vi "HandsOnCfgUI.vi"() -> ()   [LabVIEW 2013]
uses:
  <vilib>/NI/Tag Bus Data Framework/Configuration Editor/Classes/Engine Parent/Engine Parent Editor Node.lvclass
  <vilib>/NI/Tag Bus Data Framework/Configuration Editor/Classes/Module editor node/module editor node.lvclass
  <vilib>/NI/Tag Bus Data Framework/control module/editor node/control module editor.lvclass
  <vilib>/NI/Tools/Keyed Array/KeyedArray.ctl
  <vilib>/NI/Tools/Keyed Array/Tools_KeyedArray.lvlib
  <vilib>/NI/AMC/Message.ctl
  <vilib>/NI/AMC/AMC.lvlib
  <vilib>/NI/AMC/Message Queue.ctl
  <vilib>/NI/Configuration Framework/Node/NISE_CEF_Node.lvclass
  <vilib>/NI/Configuration Framework/Node/NodeRef.ctl
  <vilib>/NI/Configuration Framework/Controls/EventCluster.ctl
  <vilib>/NI/Configuration Framework/NISE_CEF_TreeControl.lvlib
  <vilib>/NI/Configuration Framework/Node/UserEventRef.ctl
  <vilib>/NI/Configuration Framework/Node/RefreshUIEvent.ctl
  <vilib>/NI/Configuration Framework/Node/CacheState.ctl
  <vilib>/NI/Configuration Framework/Node/StopEvent.ctl
  <vilib>/NI/Configuration Framework/Node/NodeChangeEvent.ctl
panel:
  in  "output range low":dbl
  in  "output range high":dbl
  in  "Output mappings":cluster{"fan":string, "lamp":string}
  in  "Input mappings":T1
  in  "node change":T2
  in  "stop event":T3
  in  "cache state":T4
  in  "refresh UI":T5
  in  "user event":T6
  in  "main queue":T7
  in  "node ref":T8
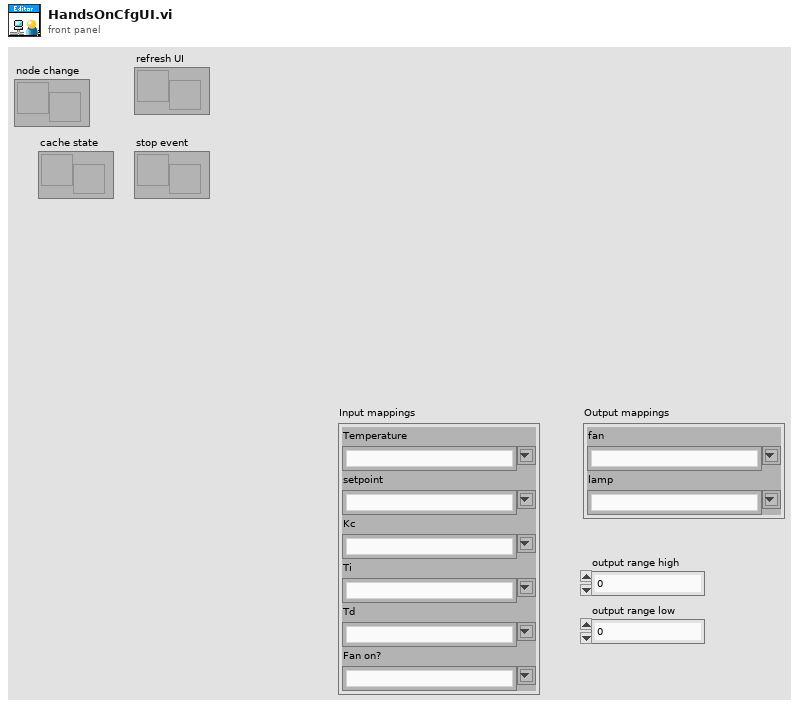
[diagram p1: front panel]
types:
  T1 = cluster{"Temperature":string, "setpoint":string, "Kc":string, "Ti":string, "Td":string, "Fan on?":string}
  T2 = typedef "NISE_CEF_Node.lvclass/NodeChangeEvent.ctl" = refnum<user-event>
  T3 = typedef "NISE_CEF_Node.lvclass/StopEvent.ctl" = refnum<user-event>
  T4 = typedef "NISE_CEF_Node.lvclass/CacheState.ctl" = refnum<user-event>
  T5 = typedef "NISE_CEF_Node.lvclass/RefreshUIEvent.ctl" = refnum<user-event>
  T6 = typedef "NISE_CEF_Node.lvclass/UserEventRef.ctl" = refnum<user-event>
  T7 = typedef "AMC.lvlib/Message Queue.ctl" = refnum<queue>
  T8 = typedef "NISE_CEF_Node.lvclass/NodeRef.ctl" = refnum<data-value>
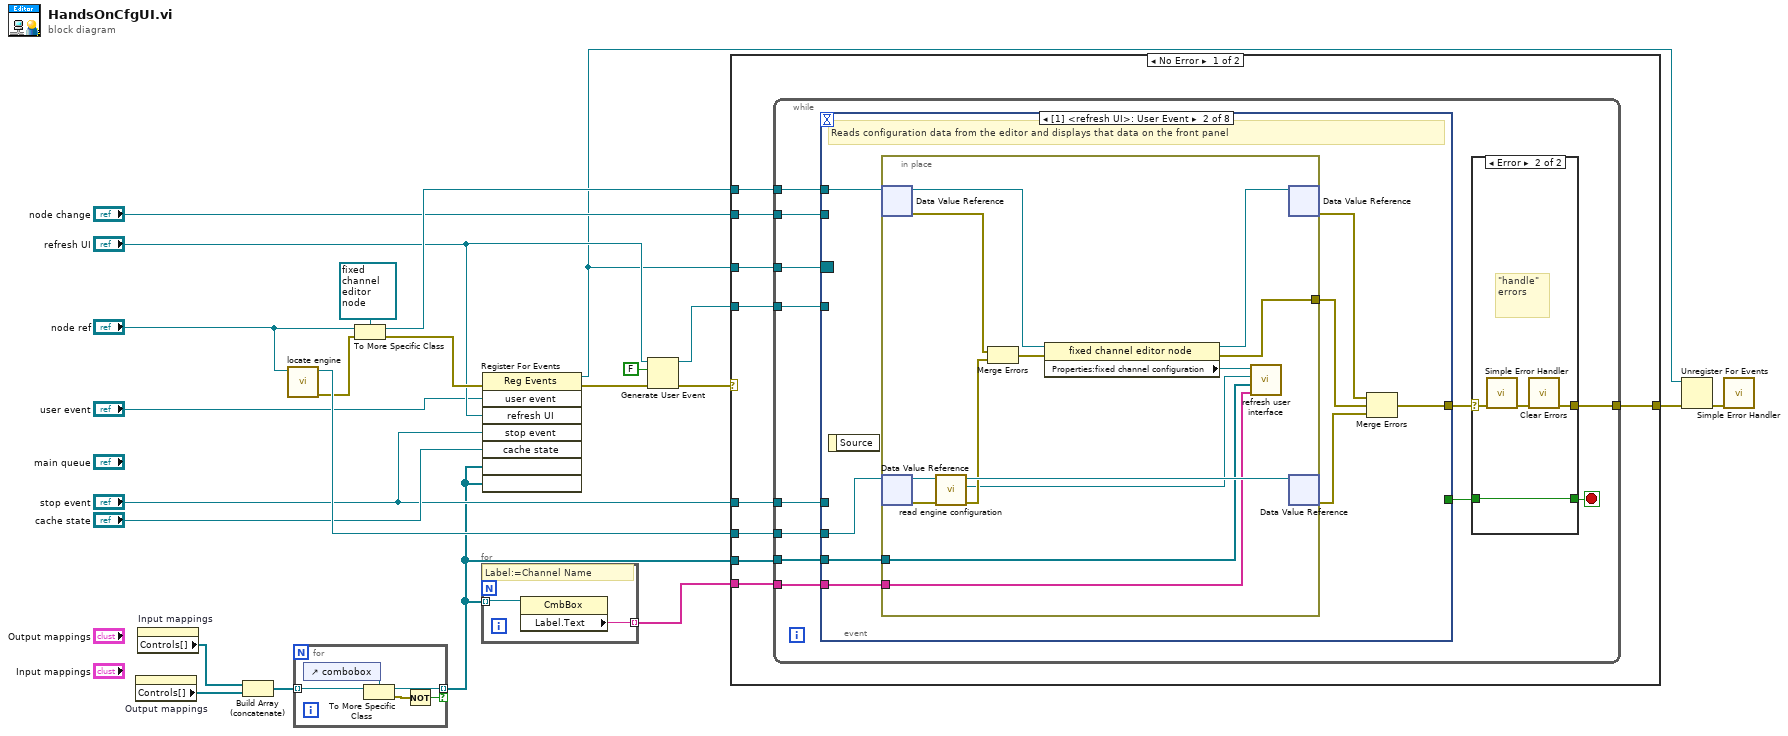
[diagram p0: block diagram]
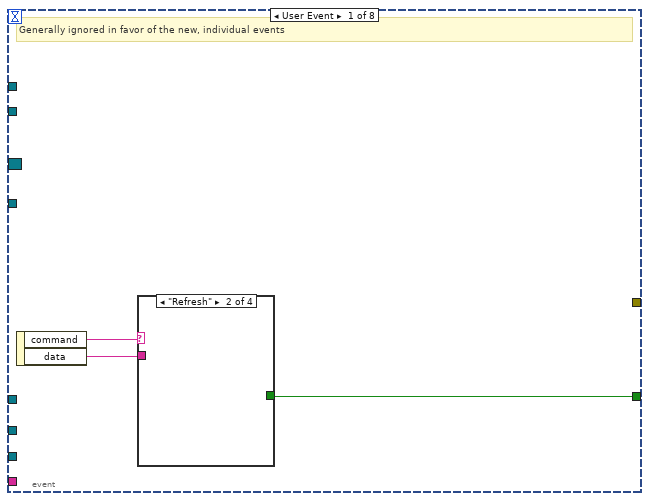
[diagram p3: hidden frame]
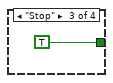
[diagram p5: hidden frame]
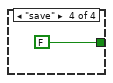
[diagram p6: hidden frame]
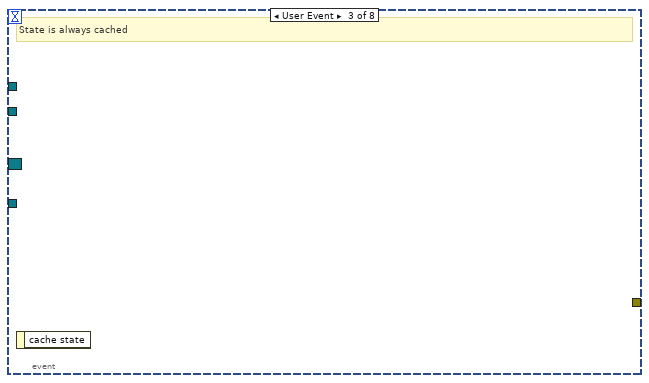
[diagram p7: hidden frame]
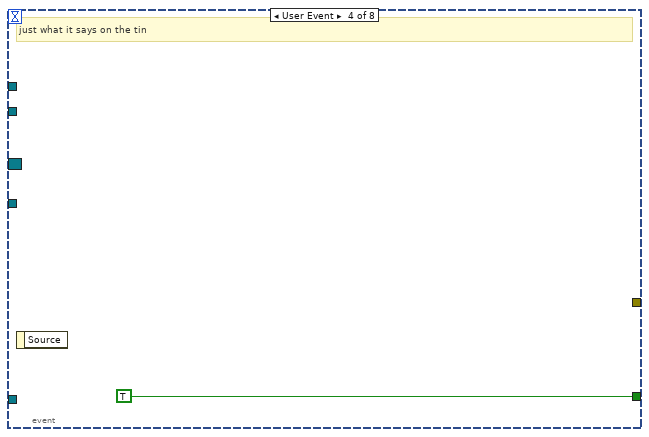
[diagram p8: hidden frame]
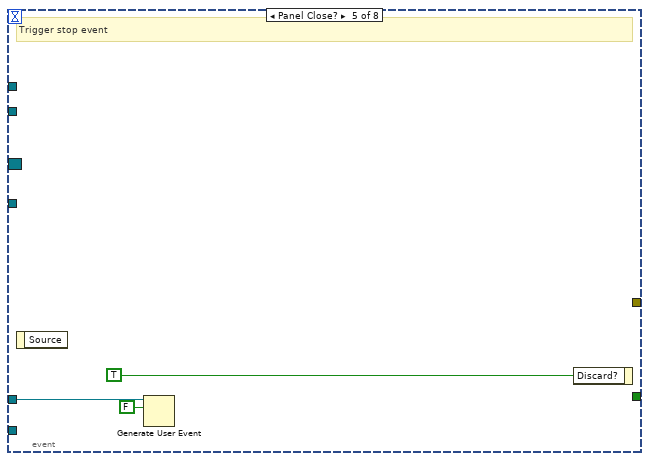
[diagram p9: hidden frame]
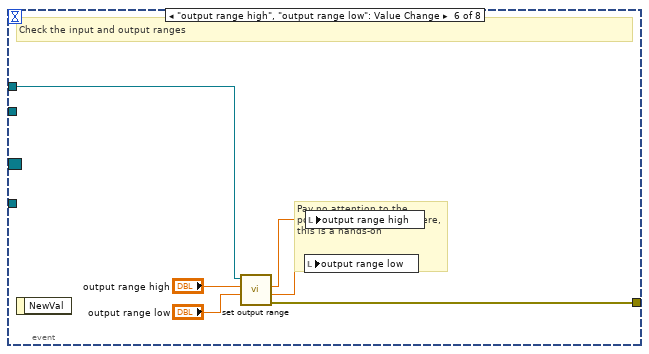
[diagram p10: hidden frame]
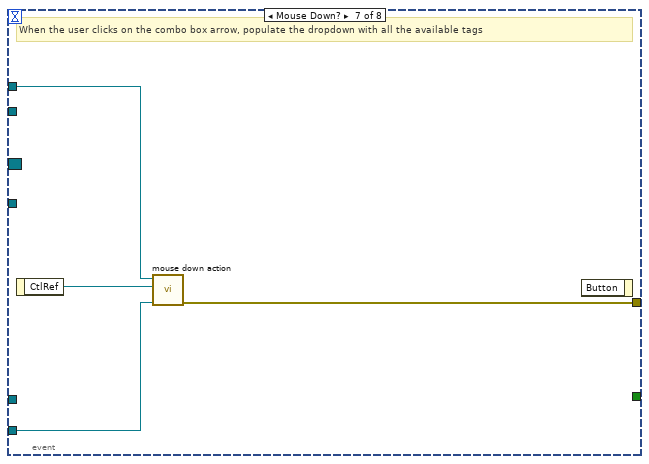
[diagram p11: hidden frame]
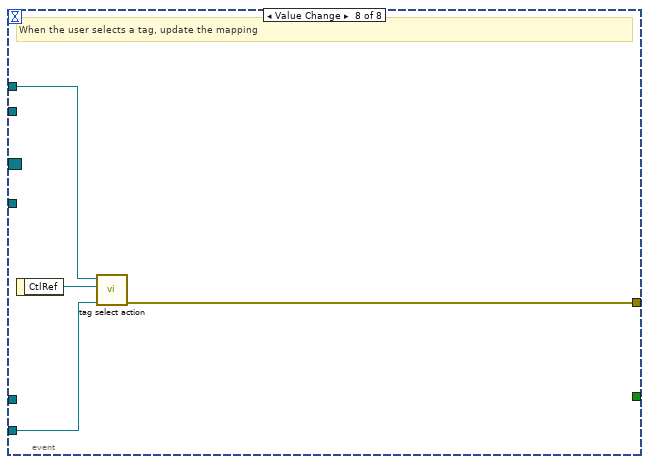
[diagram p12: hidden frame]
diagram:
  n1 = property on="Output mappings" class="Clust (strict)"() -> ("Controls[]"=w5:refnum<vi>[])  [unwired: 2 in, 2 out]
  n2 = property on="Input mappings" class="Clust (strict)"() -> ("Controls[]"=w6:refnum<vi>[])  [unwired: 2 in, 2 out]
  n3 = Build Array (concatenate)(w6, w5) -> (w3:refnum<vi>[])
  n4 = call <vilib>:"locate engine.vi"("component"="node ref") -> ("error out"=w15:errorcluster, "engine"=w17:refnum<data-value>)  [unwired: 9 in]
  n5 = for {
    tunnel: [w27] -> w1 mode=indexing if=w25
    tunnel: w3 -> [w28] mode=indexing
    n6 = control-ref of="combobox"() -> (w24:refnum<vi>)
    n7 = To More Specific Class(target class=w24, reference=w28) -> (specific class reference=w27:refnum<vi>, error out=w26:errorcluster)  [unwired: 1 in]
    n8 = Not(x=w26) -> (.not. x?=w25:bool)
  }
  n9 = To More Specific Class(target class=refnum<data-value> refnum ("data value reference"), reference="node ref", error in=w15) -> (specific class reference=w19:refnum<data-value>, error out=w18:errorcluster)
  n10 = for {
    tunnel: [w30] -> w4 mode=indexing
    tunnel: w1 -> [w29] mode=indexing
    # "Label:=Channel Name"
    n11 = property class="CmbBox"(reference=w29) -> ("Label.Text"=w30:string)  [unwired: 1 in, 2 out]
  }
  n12 = register-events(error in=w18, "user event", "refresh UI", "stop event", "cache state", w1, w1) -> (reference out=w2:refnum<event-registration>, error out=w21:errorcluster)  [unwired: 1 in]
  n13 = Generate User Event(user event="refresh UI", event data cluster=FALSE ("event data"), error in=w21) -> (user event out=w10:T5, error out=w14:errorcluster)  [unwired: 1 in]
  n14 = case shown="No Error" w14 {
    selector: w14 -> [_ w102]
    tunnel: w2 -> [w39 _]
    tunnel: [w36 w102] -> w23
    tunnel: w17 -> [w38 _]
    tunnel: w19 -> [w37 _]
    tunnel: "node change" -> [w35 _]
    tunnel: w10 -> [w34 _]
    tunnel: "stop event" -> [w33 _]
    tunnel: w1 -> [w32 _]
    tunnel: w4 -> [w31 _]
    frame No Error {
      n15 = while {
        tunnel: w39 -> [w51]
        tunnel: w37 -> [w48]
        tunnel: w38 -> [w47]
        tunnel: [w45] -> w36
        tunnel: w35 -> [w44]
        tunnel: w34 -> [w43]
        tunnel: w33 -> [w42]
        tunnel: w32 -> [w41]
        tunnel: w31 -> [w40]
        stop <- w49 stop-if-true
        n16 = event shown="[1] <refresh UI>: User Event" {
          selector: w51 -> [_ _ _ _ _ _ _ _]
          dyn-events: _ -> [_ _ _ _ _ _ _ _]
          timeout: _ -> [_ _ _ _ _ _ _ _]
          tunnel: [w60 _ _ TRUE _ _ _ _] -> w46
          tunnel: [_ w66 _ _ _ w92 w96 w100] -> w50
          tunnel: w48 -> [_ w69 _ _ _ w93 w97 w101]
          tunnel: w47 -> [_ w70 _ _ _ _ w94 w98]
          tunnel: w44 -> [_ _ _ _ _ _ _ _]
          tunnel: w43 -> [_ _ _ _ _ _ _ _]
          tunnel: w42 -> [_ _ _ _ w86 _ _ _]
          tunnel: w41 -> [_ w64 _ _ _ _ _ _]
          tunnel: w40 -> [_ w63 _ _ _ _ _ _]
          event User Event {
            # "Generally ignored in favor of the new, individual events"
            n17 = event-data() -> ("command"=w59:string, "data"=w58:string)  [unwired: 1 in]
            n18 = case shown="\"Refresh\"" w59 {
              tunnel: [_ _ TRUE FALSE] -> w60
              tunnel: w58 -> [_ _ _ _]
              frame Default {
              }
              frame "Refresh" {
              }
              frame "Stop" {
              }
              frame "save" {
              }
            }
          }
          event User Event {
            # "Reads configuration data from the editor and displays that data on the front panel"
            n19 = event-data() -> ()  [unwired: 1 in, 1 out]
            n20 = in-place {
              in-place-border: [w74] -> w65
              in-place-border: w64 -> [w71]
              in-place-border: w63 -> [w72]
              n21 = in-place-dvr #1(w69) -> (w77:refnum<class "control module editor.lvclass">, w83:errorcluster)
              n22 = in-place-dvr #2(w70) -> (w82:refnum<class "Engine Parent Editor Node.lvclass">, w81:errorcluster)
              n23 = call <vilib>:"read engine configuration.vi"("error in"=w81, "Engine Parent Editor Node in"=w82) -> ("error out"=w79:errorcluster, "engine configuration"=w73:refnum<class "engine configuration.lvclass">, "Engine Parent Editor Node out"=w80:refnum<class "Engine Parent Editor Node.lvclass">)  [unwired: 7 in]
              n24 = Merge Errors(w83, w79) -> (w78:errorcluster)
              n25 = property class="fixed channel editor node"(reference=w77, error in=w78) -> (reference out=w76:refnum<class "control module editor.lvclass">, error out=w74:errorcluster, "Properties:fixed channel configuration"=w75:refnum<class "control module configuration.lvclass">)
              n26 = call "refresh user interface.vi"("channel names (combo box labels)"=w72, "combo box references"=w71, "engine configuration"=w73, "control module configuration in"=w75) -> ()  [unwired: 8 in]
              n27 = in-place-dvr #1(w76) -> (w67:errorcluster)  [unwired: 1 out]
              n28 = in-place-dvr #2(w80) -> (w68:errorcluster)  [unwired: 1 out]
            }
            n29 = Merge Errors(w67, w65, w68) -> (w66:errorcluster)
          }
          event User Event {
            # "State is always cached"
            n30 = event-data() -> ()  [unwired: 1 in, 1 out]
          }
          event User Event {
            # "just what it says on the tin"
            n31 = event-data() -> ()  [unwired: 1 in, 1 out]
          }
          event Panel Close? {
            # "Trigger stop event"
            n32 = event-data() -> ()  [unwired: 1 in, 1 out]
            n33 = Generate User Event(user event=w86, event data cluster=FALSE ("event data")) -> ()  [unwired: 2 in, 2 out]
            n34 = event-data("Discard?"=TRUE) -> ()  [unwired: 1 in, 1 out]
          }
          event "output range high", "output range low": Value Change {
            # "Pay no attention to the potential race condition here, this is a hands-on"
            # "Check the input and output ranges"
            n35 = event-data() -> ()  [unwired: 1 in, 1 out]
            n36 = call "set output range.vi"("output range low (requested)"="output range low", "output range high (requested)"="output range high", "module editor in"=w93) -> ("error out"=w92:errorcluster, "output range low (real)"=w89:dbl, "output range high (real)"=w88:dbl)  [unwired: 6 in]
            n37 = local write "output range low"(w89) -> ()
            n38 = local write "output range high"(w88) -> ()
          }
          event Mouse Down? {
            # "When the user clicks on the combo box arrow, populate the dropdown with all the available tags"
            n39 = event-data() -> ("CtlRef"=w95:refnum<vi>)  [unwired: 1 in]
            n40 = call "mouse down action.vi"("engine"=w94, "CtlRef"=w95, "module editor reference"=w97) -> ("error out"=w96:errorcluster)  [unwired: 8 in]
            n41 = event-data() -> ()  [unwired: 2 in, 1 out]
          }
          event Value Change {
            # "When the user selects a tag, update the mapping"
            n42 = event-data() -> ("CtlRef"=w99:refnum<vi>)  [unwired: 1 in]
            n43 = call "tag select action.vi"("engine"=w98, "CtlRef"=w99, "module editor"=w101) -> ("error out"=w100:errorcluster)  [unwired: 8 in]
          }
        }
        n44 = case shown="Error" w50 {
          selector: w50 -> [w52 w55]
          tunnel: [w53 w57] -> w49
          tunnel: w46 -> [w53 w57]
          tunnel: [w52 w56] -> w45
          frame No Error {
          }
          frame Error {
            # "\"handle\" errors"
            n45 = call <vilib>:"Simple Error Handler.vi"("error in (no error)"=w55) -> ("error out"=w54:errorcluster)  [unwired: 4 in, 4 out]
            n46 = call <vilib>:"Clear Errors.vi"("error in (no error)"=w54) -> ("error out"=w56:errorcluster)  [unwired: 5 in, 1 out]
          }
        }
      }
    }
    frame Error {
    }
  }
  n47 = Unregister For Events(event registration refnum=w2, error in=w23) -> (error out=w20:errorcluster)
  n48 = call <vilib>:"Simple Error Handler.vi"("error in (no error)"=w20) -> ()  [unwired: 4 in, 5 out]
